vi "串口发送.vi"(6 "写入缓冲区":string, 7 "命令":string(combo), 8 "error in (no error)":errorcluster caption="错误输入（无错误）", 10 "baud rate (9600)":u32=115200 caption="波特率(115200)", 11 "VISA resource name":refnum<visa-resource-name> caption="VISA资源名称") -> (0 "错误输出":errorcluster, 3 "VISA resource name 2":refnum<visa-resource-name>, 4 "读取缓冲区":string)   [LabVIEW 2016, in "数据传输系统.lvlib"]
uses:
  <vilib>/Instr/_visa.llb/VISA Flush IO Buffer Mask.ctl
  <vilib>/Instr/_visa.llb/VISA Configure Serial Port (Instr).vi
panel:
  in  "timeout (10sec)":u32=10000 caption="超时（10秒）"
  out "返回数":u32
  in  "parity (0:none)":enum16{"None", "Odd", "Even", "Mark", "Space"}(ring) caption="奇偶（0:无）"
  in  "data bits (8)":u16=8 caption="数据比特(8)" min=5 max=8 step=1
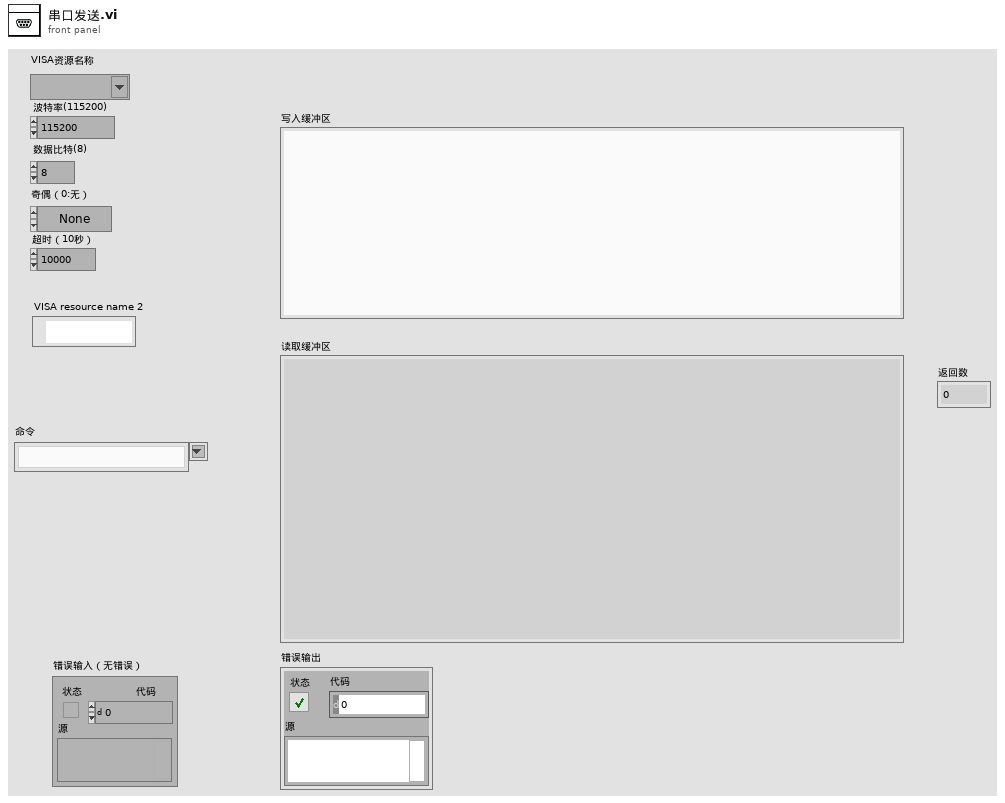
[diagram p1: front panel]
types:
  T1 = typedef "VISA Flush IO Buffer Mask.ctl" = u16
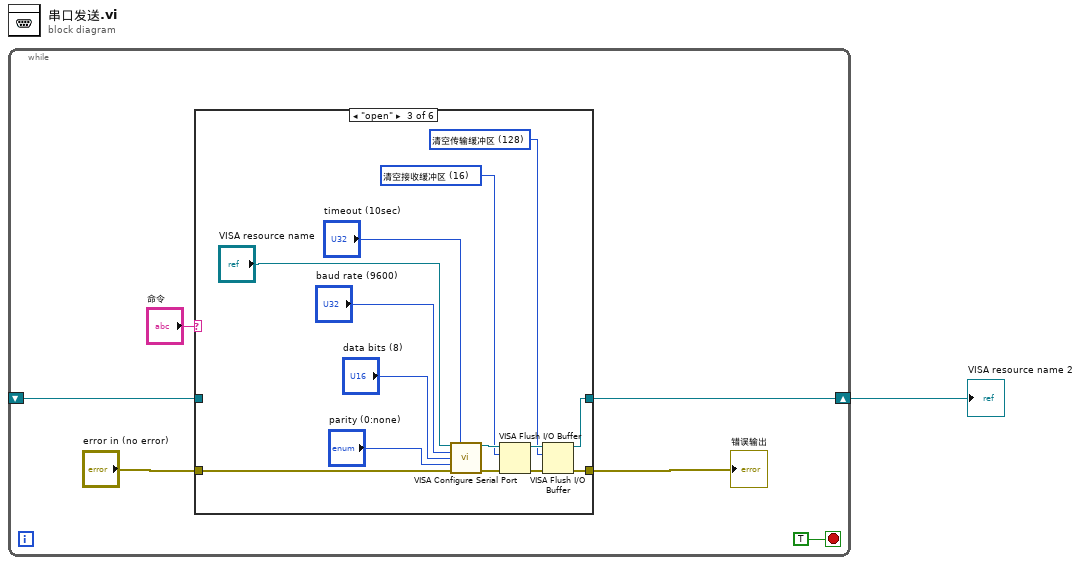
[diagram p0: block diagram]
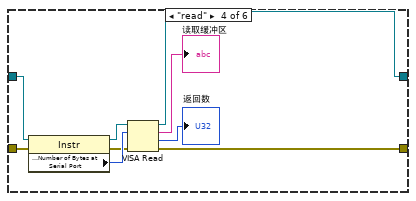
[diagram p4: hidden frame]
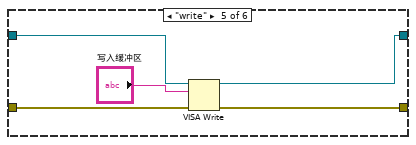
[diagram p5: hidden frame]
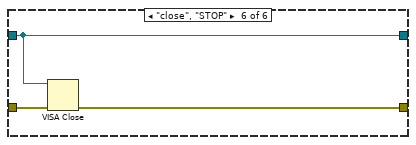
[diagram p6: hidden frame]
diagram:
  n1 = while {
    shift-right: [w4] -> w1
    shift-left: _ -> [w2]
    stop <- TRUE stop-if-true
    n2 = case shown="\"open\"" "命令" {
      tunnel: "error in (no error)" -> [w9 w11 w22 w33 w38 w42]
      tunnel: [w9 w11 w14 w27 w37 w41] -> w6
      tunnel: w2 -> [w8 w10 _ w34 w39 w40]
      tunnel: [w8 w10 w13 w26 w35 w40] -> w4
      frame "idle", Default {
      }
      frame "init" {
      }
      frame "open" {
        w15 = T1 128 items=["清空接收缓冲区"=16, "向设备写入传输缓冲区"=32, "清空接收缓冲区（无I/O）"=64, "清空传输缓冲区"=128] ("Mask")
        w18 = T1 16 items=["清空接收缓冲区"=16, "向设备写入传输缓冲区"=32, "清空接收缓冲区（无I/O）"=64, "清空传输缓冲区"=128] ("Mask")
        n3 = call-poly "VISA Configure Serial Port"("VISA resource name"="VISA resource name", "timeout (10sec)"="timeout (10sec)", "baud rate (9600)"="baud rate (9600)", "data bits (8)"="data bits (8)", "parity (0:none)"="parity (0:none)", "error in (no error)"=w22) -> ("VISA resource name out"=w20:refnum<visa-resource-name>, "error out"=w21:errorcluster)  [unwired: 8 in]
        n4 = VISA Flush I/O Buffer(VISA resource name=w20, mask (16)=w18, error in (no error)=w21) -> (VISA resource name out=w16:refnum<visa-resource-name>, error out=w17:errorcluster)
        n5 = VISA Flush I/O Buffer(VISA resource name=w16, mask (16)=w15, error in (no error)=w17) -> (VISA resource name out=w13:refnum<visa-resource-name>, error out=w14:errorcluster)
      }
      frame "read" {
        n6 = property class="Instr"(reference=w34, error in=w33) -> (reference out=w30:refnum<visa-resource-name>, error out=w31:errorcluster, "Serial Settings:Number of Bytes at Serial Port"=w32:u32)
        n7 = VISA Read(VISA resource name=w30, byte count=w32, error in (no error)=w31) -> (VISA resource name out=w26:refnum<visa-resource-name>, read buffer=→"读取缓冲区":string, return count=→"返回数":u32, error out=w27:errorcluster)
      }
      frame "write" {
        n8 = VISA Write(VISA resource name=w39, write buffer="写入缓冲区", error in (no error)=w38) -> (VISA resource name out=w35:refnum<visa-resource-name>, error out=w37:errorcluster)  [unwired: 1 out]
      }
      frame "close", "STOP" {
        n9 = VISA Close(VISA resource name=w40, error in (no error)=w42) -> (error out=w41:errorcluster)
      }
    }
    "错误输出" <- w6
  }
  "VISA resource name 2" <- w1
